vi "controlMotor.vi"(8 "Mover":bool, 9 "Posición deseada":dbl, 10 "Longitud Actual":dbl, 11 "comenzar":bool) -> (3 "Posicion actual":dbl)   [LabVIEW 2013]
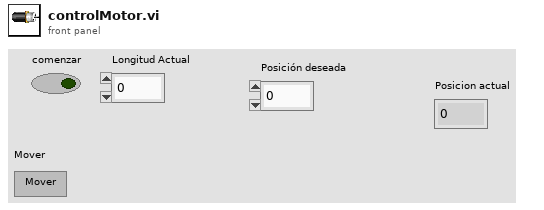
[diagram p1: front panel]
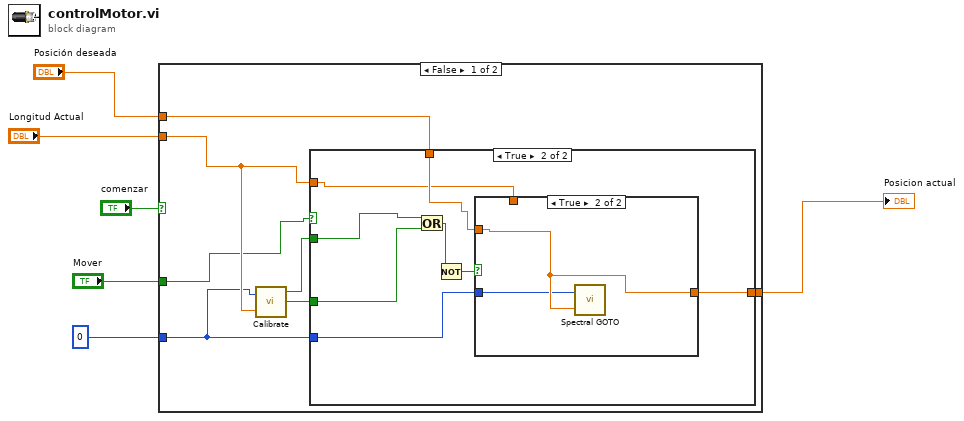
[diagram p0: block diagram]
diagram:
  n1 = case shown="False" "comenzar" {
    tunnel: "Longitud Actual" -> [w13 w26]
    tunnel: [w10 w26] -> w3
    tunnel: "Posición deseada" -> [w9 _]
    tunnel: "Mover" -> [w8 _]
    tunnel: 0 ("Spectrometer Number") -> [w7 _]
    frame False {
      n2 = call "Calibrate.VI"("Spectrometer Number"=w7, "Counter Position"=w13) -> ("Error"=w12:bool, "Invalid Wavelength"=w11:bool)  [unwired: 1 out]
      n3 = case shown="True" w8 {
        tunnel: w13 -> [w14 w16]
        tunnel: w9 -> [_ w22]
        tunnel: w12 -> [_ w19]
        tunnel: w11 -> [_ w18]
        tunnel: [w14 w17] -> w10
        tunnel: w7 -> [_ w15]
        frame False {
        }
        frame True {
          n4 = Or(x=w19, y=w18) -> (x .or. y?=w20:bool)
          n5 = Not(x=w20) -> (.not. x?=w21:bool)
          n6 = case shown="True" w21 {
            tunnel: w22 -> [_ w25]
            tunnel: [w23 w25] -> w17
            tunnel: w16 -> [w23 _]
            tunnel: w15 -> [_ w24]
            frame False {
            }
            frame True {
              n7 = call "Spectral GOTO.VI"("Spectrometer Number"=w24, "Target Position"=w25) -> ()  [unwired: 3 out]
            }
          }
        }
      }
    }
    frame True {
    }
  }
  "Posicion actual" <- w3
